vi "Send Add Expected Heartbeat.vi"(6 "Timeout":u16 format="%d ms", 7 "Message Priority (Normal)":T1=enum."Normal", 8 "error in (no error)":errorcluster, 9 "Period":u16 format="%d ms", 10 "Node-ID":u8, 11 "Message Enqueuer":refnum<class "Message Enqueuer.lvclass">) -> (0 "error out":errorcluster, 3 "Message Enqueuer out":refnum<class "Message Enqueuer.lvclass">)   [LabVIEW 2020, in "Interactor.lvlib" / "Add Expected Heartbeat Msg.lvclass"]
doc: "This VI sends the message to an actor."
uses:
  Add Expected Heartbeat Msg.lvclass
  Add Expected Heartbeat Msg.lvclass/Add Expected Heartbeat Msg.ctl
  <vilib>/ActorFramework/Message Enqueuer/Message Enqueuer.lvclass
  <vilib>/ActorFramework/Message Enqueuer/Message Priority.ctl
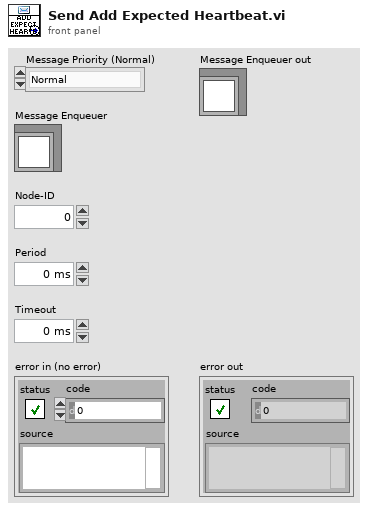
[diagram p1: front panel]
types:
  T1 = typedef "Actor Framework.lvlib/Message Enqueuer.lvclass/Message Priority.ctl" = enum16{"Low", "Normal", "High"}
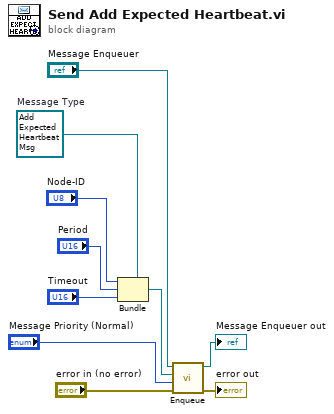
[diagram p0: block diagram]
diagram:
  w7 = refnum<class "Add Expected Heartbeat Msg.lvclass"> refnum  # Message Type
  n1 = Bundle(cluster=w7, "Node-ID", "Period", "Timeout") -> (w6:refnum<class "Add Expected Heartbeat Msg.lvclass">)
  n2 = call <vilib>:"Enqueue.vi"("error in (no error)"="error in (no error)", "Message Priority (Normal)"="Message Priority (Normal)", "Message"=w6, "Message Enqueuer in"="Message Enqueuer") -> ("error out"=→"error out":errorcluster, "Message Enqueuer out"=→"Message Enqueuer out":refnum<class "Message Enqueuer.lvclass">)  [unwired: 6 in]
